vi "REQ(HB).vi"() -> ()   [LabVIEW 2014]
uses:
  <vilib>/addons/zeromq/socket_type.ctl
  <userlib>/_OpenG.lib/numeric/numeric.llb/Random Number Within Range - DBL__ogtk.vi
  <vilib>/addons/zeromq/zmq_context.lvclass
  <vilib>/addons/zeromq/zeromq.lvlib
  <vilib>/addons/zeromq/zmq_socket.lvclass
panel:
  in  "stop":bool
  in  "Request":bool
  out "concatenated string":string
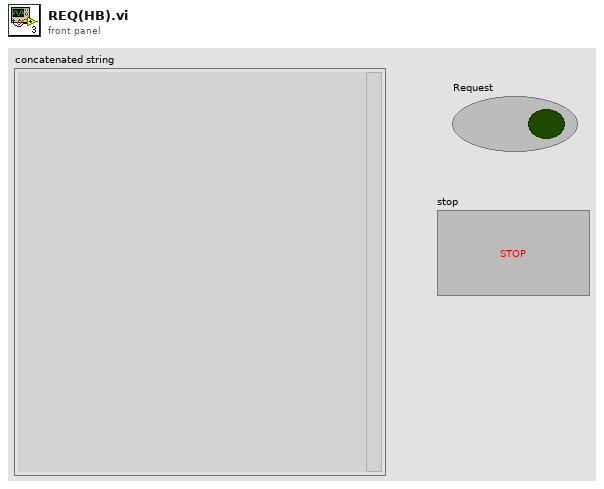
[diagram p1: front panel]
types:
  T1 = typedef "zeromq.lvlib/socket_type.ctl" = enum8{"ZMQ_PAIR", "ZMQ_PUB", "ZMQ_SUB", "ZMQ_REQ", "ZMQ_REP", "ZMQ_DEALER", "ZMQ_ROUTER", "ZMQ_PULL", "ZMQ_PUSH", "ZMQ_XPUB", "ZMQ_XSUB", "ZMQ_STREAM", "ZMQ_SERVER", "ZMQ_CLIENT", "ZMQ_RADIO", "ZMQ_DISH", "ZMQ_GATHER", "ZMQ_SCATTER", "ZMQ_DGRAM"}
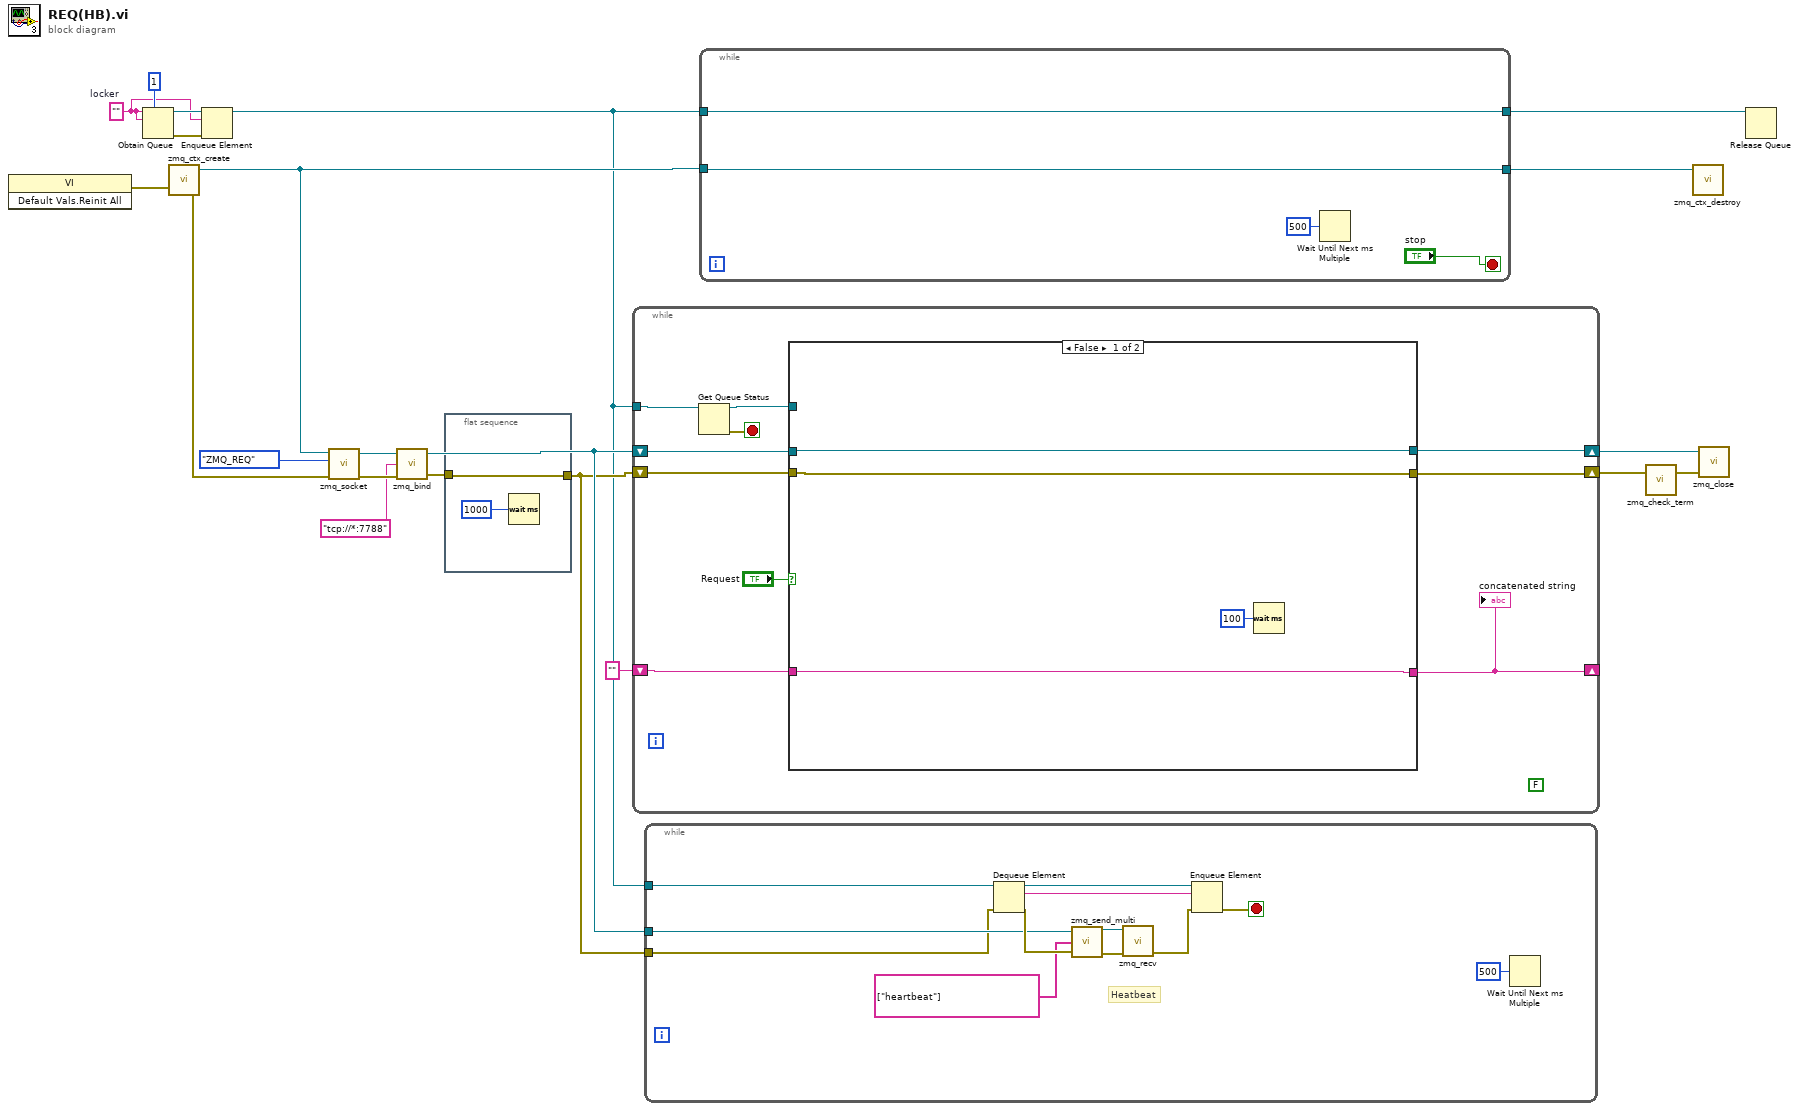
[diagram p0: block diagram]
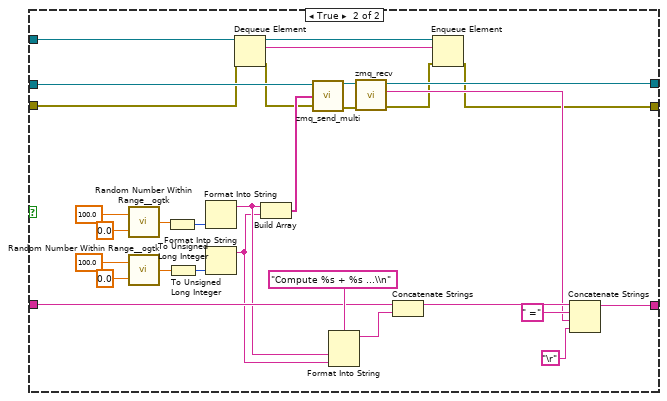
[diagram p2: hidden frame]
diagram:
  w7 = ""  # locker
  n1 = invoke class="VI" method="Default Vals.Reinit All"() -> (error out=w13:errorcluster)  [unwired: 3 in, 2 out]
  n2 = Obtain Queue(max queue size (-1, unlimited)=1, name (unnamed)=w7, element data type=w7) -> (queue out=w9:refnum<queue>, error out=w8:errorcluster)  [unwired: 2 in, 1 out]
  n3 = call <vilib>:"zmq_ctx_create.vi"("error in"=w13) -> ("error out"=w20:errorcluster, "context out"=w4:refnum<class "zmq_context.lvclass">)  [unwired: 3 in]
  n4 = Enqueue Element(queue=w9, element=w7, error in (no error)=w8) -> (queue out=w1:refnum<queue>)  [unwired: 1 in, 2 out]
  n5 = call <vilib>:"zmq_socket.vi"("error in"=w20, "socket type"=socket_type."ZMQ_REQ", "context in"=w4) -> ("error out"=w18:errorcluster, "socket out"=w19:refnum<class "zmq_socket.lvclass">)  [unwired: 2 in, 1 out]
  n6 = call <vilib>:"zmq_bind.vi"("error in"=w18, "endpoint"="tcp://*:7788", "socket in"=w19) -> ("error out"=w15:errorcluster, "socket out"=w12:refnum<class "zmq_socket.lvclass">)  [unwired: 1 in]
  n7 = flat-sequence {
    tunnel: [w22] -> w11
    tunnel: w15 -> [w22]
    frame #0 {
      n8 = Wait (ms)(milliseconds to wait=u32 1000) -> ()  [unwired: 1 out]
    }
  }
  n9 = while {
    shift-right: [w32] -> w16
    shift-left: w12 -> [w33]
    shift-right: [w27] -> w6
    shift-left: w11 -> [w31]
    shift-right: [w29] -> _
    shift-left: "" -> [w30]
    tunnel: w1 -> [w26]
    stop <- w24 stop-if-true
    (unwired) FALSE
    n10 = Get Queue Status(queue=w26) -> (queue out=w25:refnum<queue>, error out=w24:errorcluster)  [unwired: 2 in, 6 out]
    n11 = case shown="False" "Request" {
      tunnel: w33 -> [w36 w67]
      tunnel: [w36 w64] -> w32
      tunnel: [w35 w38] -> w27
      tunnel: w31 -> [w35 w40]
      tunnel: w30 -> [w37 w52]
      tunnel: [w37 w48] -> w29
      tunnel: w25 -> [_ w44]
      frame False {
        n12 = Wait (ms)(milliseconds to wait=u32 100) -> ()  [unwired: 1 out]
      }
      frame True {
        n13 = call-poly <userlib>:"Random Number Within Range__ogtk.vi"("High"=100.0, "Low"=0.0) -> ("Random Number"=w59:dbl)  [unwired: 3 in]
        n14 = call-poly <userlib>:"Random Number Within Range__ogtk.vi"("High"=100.0, "Low"=0.0) -> ("Random Number"=w58:dbl)  [unwired: 3 in]
        n15 = To Unsigned Long Integer(number=w59) -> (unsigned 32bit integer=w57:u32)
        n16 = To Unsigned Long Integer(number=w58) -> (unsigned 32bit integer=w56:u32)
        n17 = Format Into String(w57) -> (resulting string=w51:string)  [unwired: 3 in, 1 out]
        n18 = Format Into String(w56) -> (resulting string=w50:string)  [unwired: 3 in, 1 out]
        n19 = Dequeue Element(queue=w44, error in (no error)=w40) -> (queue out=w43:refnum<queue>, element=w42:string, error out=w41:errorcluster)  [unwired: 1 in, 1 out]
        n20 = Build Array(w51, w50) -> (w55:string[])
        n21 = call <vilib>:"zmq_send_multi.vi"("error in"=w41, "parts"=w55, "socket in"=w67) -> ("error out"=w66:errorcluster, "socket out"=w65:refnum<class "zmq_socket.lvclass">)  [unwired: 1 in]
        n22 = Format Into String(format string="Compute %s + %s ...\\n", w51, w50) -> (resulting string=w54:string)  [unwired: 2 in, 1 out]
        n23 = call <vilib>:"zmq_recv.vi"("error in"=w66, "socket in"=w65) -> ("error out"=w39:errorcluster, "data"=w46:string, "socket out"=w64:refnum<class "zmq_socket.lvclass">)  [unwired: 3 in, 2 out]
        n24 = Concatenate Strings(w52, w54) -> (w49:string)
        n25 = Enqueue Element(queue=w43, element=w42, error in (no error)=w39) -> (error out=w38:errorcluster)  [unwired: 1 in, 2 out]
        n26 = Concatenate Strings(w49, " =" ("string"), w46, "\r") -> (w48:string)
      }
    }
    "concatenated string" <- w29
  }
  n27 = while {
    tunnel: w12 -> [w72]
    tunnel: w11 -> [w71]
    tunnel: w1 -> [w70]
    stop <- w68 stop-if-true
    # "Heatbeat"
    n28 = Dequeue Element(queue=w70, error in (no error)=w71) -> (queue out=w75:refnum<queue>, element=w76:string, error out=w77:errorcluster)  [unwired: 1 in, 1 out]
    n29 = call <vilib>:"zmq_send_multi.vi"("error in"=w77, "parts"=string[] ["heartbeat"], "socket in"=w72) -> ("error out"=w73:errorcluster, "socket out"=w74:refnum<class "zmq_socket.lvclass">)  [unwired: 1 in]
    n30 = call <vilib>:"zmq_recv.vi"("error in"=w73, "socket in"=w74) -> ("error out"=w78:errorcluster)  [unwired: 3 in, 4 out]
    n31 = Enqueue Element(queue=w75, element=w76, error in (no error)=w78) -> (error out=w68:errorcluster)  [unwired: 1 in, 2 out]
    n32 = Wait Until Next ms Multiple(millisecond multiple=u32 500 ("milliseconds to wait")) -> ()  [unwired: 1 out]
  }
  n33 = while {
    tunnel: w4 -> [w83]
    tunnel: [w83] -> w3
    tunnel: [w82] -> w2
    tunnel: w1 -> [w82]
    stop <- "stop" stop-if-true
    n34 = Wait Until Next ms Multiple(millisecond multiple=u32 500 ("milliseconds to wait")) -> ()  [unwired: 1 out]
  }
  n35 = call <vilib>:"zmq_check_term.vi"("error in"=w6) -> ("error out"=w5:errorcluster)  [unwired: 1 in, 1 out]
  n36 = call <vilib>:"zmq_ctx_destroy.vi"("context in"=w3) -> ()  [unwired: 4 in, 1 out]
  n37 = call <vilib>:"zmq_close.vi"("error in"=w5, "socket"=w16) -> ()  [unwired: 3 in, 1 out]
  n38 = Release Queue(queue=w2) -> ()  [unwired: 2 in, 3 out]
